vi "Tag Create.vi"(8 "Data":variant, 9 "Data Count":u32=1, 10 "Data Type":T1(ring)=enum."U16", 11 "Tag ID":u16) -> (3 "IFD_Tag out":refnum<class "IFD_Tag.lvclass">)   [LabVIEW 2016, in "IFD_Tag.lvclass"]
uses:
  IFD_Tag.lvclass
  IFD_Tag.lvclass/IFD_Tag.ctl
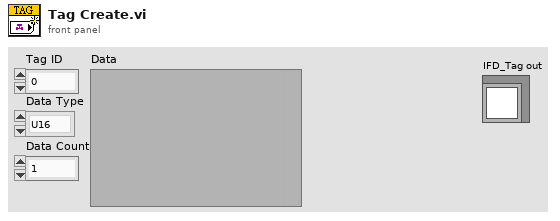
[diagram p1: front panel]
types:
  T1 = enum16{"Undefined(DO NOT USE)", "U8", "ASCII", "U16", "U32", "RATIONAL", "I8", "Undefined 8 bit", "I16", "I32", "SRATIONAL", "SGL", "DBL"}
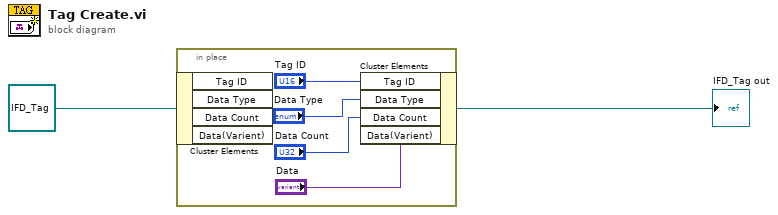
[diagram p0: block diagram]
diagram:
  n1 = in-place {
    n2 = in-place-cluster #1(refnum<class "IFD_Tag.lvclass"> refnum ("IFD_Tag.lvclass")) -> ()  [unwired: 4 out]
    n3 = in-place-cluster #1("Tag ID"="Tag ID", "Data Type"="Data Type", "Data Count"="Data Count", "Data(Varient)"="Data") -> (→"IFD_Tag out":refnum<class "IFD_Tag.lvclass">)
  }
